vi "Read Command Queue.vi"(8 "error in (no error)":errorcluster, 11 "Command Processor Actor in":refnum<class "Command Processor Actor.lvclass">) -> (0 "error out":errorcluster, 2 "Queued Commands":refnum<queue>, 3 "Command Processor Actor out":refnum<class "Command Processor Actor.lvclass">)   [LabVIEW 2014, in "Robot Actor Framework.lvlib" / "Command Processor Actor.lvlib" / "Command Processor Actor.lvclass"]
uses:
  Command Processor Actor.lvclass
  Command Actor/Command Actor Class/Command Actor.lvclass
  Command Processor Actor.lvclass/Command Processor Actor.ctl
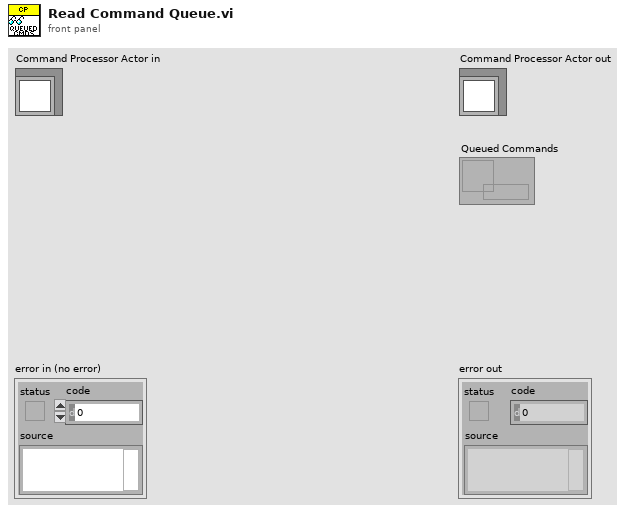
[diagram p1: front panel]
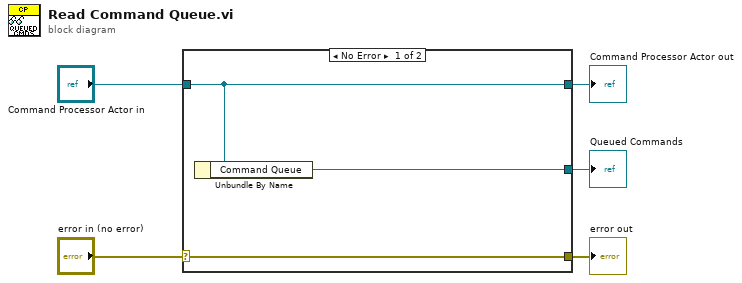
[diagram p0: block diagram]
diagram:
  n1 = case shown="No Error" "error in (no error)" {
    selector: "error in (no error)" -> [w8 w9]
    tunnel: [w8 w9] -> w4
    tunnel: [w7 w10] -> w2
    tunnel: "Command Processor Actor in" -> [w7 w10]
    tunnel: [w6 _] -> w1
    frame No Error {
      n2 = Unbundle By Name(w7) -> ("Command Queue"=w6:refnum<queue>)
    }
    frame Error {
    }
  }
  "error out" <- w4
  "Command Processor Actor out" <- w2
  "Queued Commands" <- w1
